vi "PFI-28000-Utils_String Contains.vi"(0 "String":string, 5 "Value":string) -> (4 "Match":string, 6 "After Substring":string, 8 "Contains":bool)   [LabVIEW 2017, in "PFI-28000-Utils.lvlib"]
uses:
  PFI-28000-Utils.lvlib
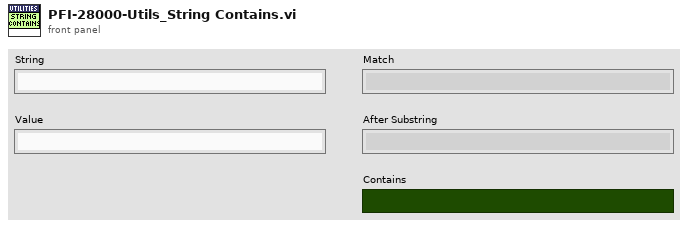
[diagram p1: front panel]
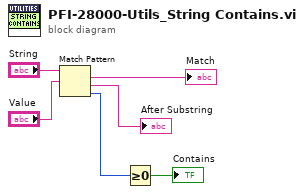
[diagram p0: block diagram]
diagram:
  n1 = Match Pattern(string="String", regular expression="Value") -> (match substring=→"Match":string, after substring=→"After Substring":string, offset past match=w6:i32)  [unwired: 1 in, 1 out]
  n2 = Greater Or Equal To 0?(x=w6) -> (x >= 0?=→"Contains":bool)
